vi "XNET Read (Signal Single-point).vi"(0 "session in":refnum<k21>, 11 "error in (no error)":errorcluster) -> (4 "session out":refnum<k21>, 6 "data":dbl[](array[numeric]) format="%.2f", 15 "error out":errorcluster)   [LabVIEW 2018]
doc: "Reads data from a session of Signal Input Single-Point mode."
uses:
  nixlvapi.dll
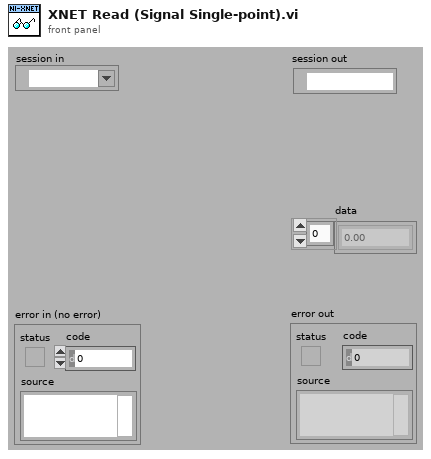
[diagram p1: front panel]
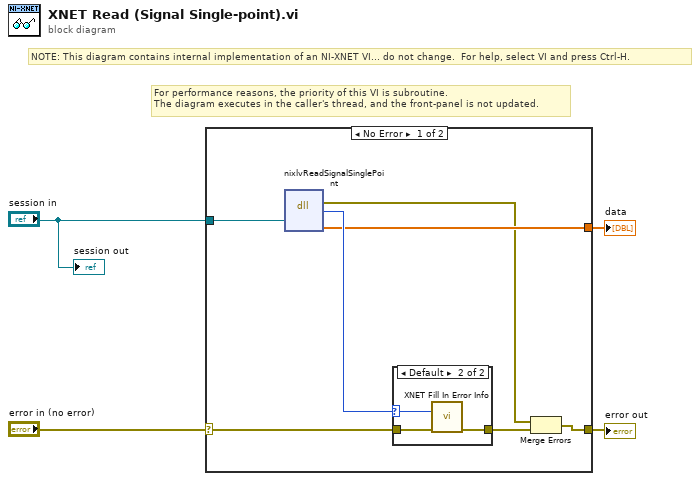
[diagram p0: block diagram]
diagram:
  # "For performance reasons, the priority of this VI is subroutine.\nThe diagram executes in the caller's thread, and the front-panel is not updated."
  # "NOTE: This diagram contains internal implementation of an NI-XNET VI... do not change.  For help, select VI and press Ctrl-H."
  n1 = case shown="No Error" "error in (no error)" {
    selector: "error in (no error)" -> [w9 w16]
    tunnel: "session in" -> [w11 _]
    tunnel: [w6 w16] -> w4
    tunnel: [w7 _] -> w1
    frame No Error {
      n2 = dll-call lib="nixlvapi.*" fn="nixlvReadSignalSinglePoint"("sessionRef"=w11) -> (error out=w5:errorcluster, "return type"=w8:i32, "lvData"=w7:dbl[])  [unwired: 3 in, 3 out]
      n3 = case shown="Default" w8 {
        selector: w8 -> [_ w13]
        tunnel: w9 -> [w12 w14]
        tunnel: [w12 w15] -> w10
        frame 0 {
        }
        frame Default {
          n4 = call "XNET Fill In Error Info.vi"("status code"=w13, "error in"=w14) -> ("error out"=w15:errorcluster)  [unwired: 13 out]
        }
      }
      n5 = Merge Errors(w5, w10) -> (w6:errorcluster)
    }
    frame Error {
    }
  }
  "error out" <- w4
  "data" <- w1
  "session out" <- "session in"
